vi "saveAndClose.vi"   [LabVIEW 2015]
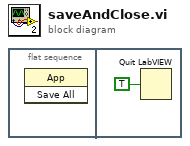
[diagram p0: block diagram]
diagram:
  n1 = flat-sequence {
    frame #0 {
      n2 = invoke class="App" method="Save All"() -> ()  [unwired: 3 in, 3 out]
    }
    frame #1 {
      n3 = Quit LabVIEW(quit? (T)=TRUE) -> ()
    }
  }
